vi "main.vi"() -> ()   [LabVIEW 2019]
uses:
  <vilib>/Utility/sysdir.llb/System Directory Type.ctl
  <vilib>/LabVIEW Open Source Project/MQTT Client/Client class/Client.lvclass/Client.ctl
  <vilib>/LabVIEW Open Source Project/MQTT Connection/MQTT_Base/Base Class/MQTT_Base.lvclass/MQTT_Base.ctl
  <vilib>/LabVIEW Open Source Project/MQTT Control Packets/Control Packets/ControlPacket/QualityOfService -- enum.ctl
  <vilib>/LabVIEW Open Source Project/MQTT Control Packets/Control Packets/ControlPacket/ControlPacket.lvclass/ControlPacket.ctl
  <vilib>/LabVIEW Open Source Project/MQTT Control Packets/Control Packets/CONNECT/ConnectFlags -- cluster.ctl
  <vilib>/LabVIEW Open Source Project/Connection/Connection.TCP/Connection.TCP.lvclass
  C:/Program Files (x86)/National Instruments/LabVIEW 2019/vi.lib/LabVIEW Open Source Project/Connection/Connection/Connection.lvclass
  <vilib>/LabVIEW Open Source Project/MQTT Client/Client class/Client.lvclass
  C:/Program Files (x86)/National Instruments/LabVIEW 2019/vi.lib/LabVIEW Open Source Project/MQTT Connection/MQTT_Base/Base Class/MQTT_Base.lvclass
  <vilib>/LabVIEW Open Source Project/MQTT Control Packets/Control Packets/PUBLISH/PUBLISH.lvclass
  C:/Program Files (x86)/National Instruments/LabVIEW 2019/vi.lib/LabVIEW Open Source Project/MQTT Control Packets/Control Packets/ControlPacket/ControlPacket.lvclass
  <vilib>/LabVIEW Open Source Project/MQTT Connection/MQTT_Base/Base Class/MQTT_Base.lvclass
  <vilib>/LabVIEW Open Source Project/MQTT Control Packets/Control Packets/ControlPacket/ControlPacket.lvclass
  <vilib>/LabVIEW Open Source Project/MQTT Control Packets/Control Packets/CONNECT/CONNECT.lvclass
  <vilib>/LabVIEW Open Source Project/Connection/Connection.LocalQueue/Connection.LocalQueue.lvclass
  <vilib>/LabVIEW Open Source Project/Connection/Connection/Connection.lvclass
panel:
  out "msg":string
  in  "publish":bool
  out "mac":string
  out "last error":errorcluster
  out "Database":bool
  out "Time Stamp Control":timestamp format="%<%X\n%x>T"
  in  "Tab Control":T1(tab)
  in  "Listbox":i32(listbox)
  in  "Users allowed per Node":u16(ring) items=["Veiculo QXC-01"]
  in  "Add Button":bool
  in  "Nodes":i32(listbox)
  in  "Users":i32(listbox)
  out "Users":dbl
  out "Nodes":dbl
  in  "Employee List":i32(listbox)
  in  "Nodes Esp32":i32(listbox)
  in  "Broker Port":dbl=1883.0
  in  "Broker Address":string="broker.hivemq.com"
  in  "Connection":bool
  in  "Subscribe":bool
  in  "Settings Button":bool
  in  "Payroll Button":bool
  in  "Logs Button":bool
  in  "Nodes Button":bool
  in  "Employee Button":bool
  in  "Home Button":bool
  # "COMING SOON"
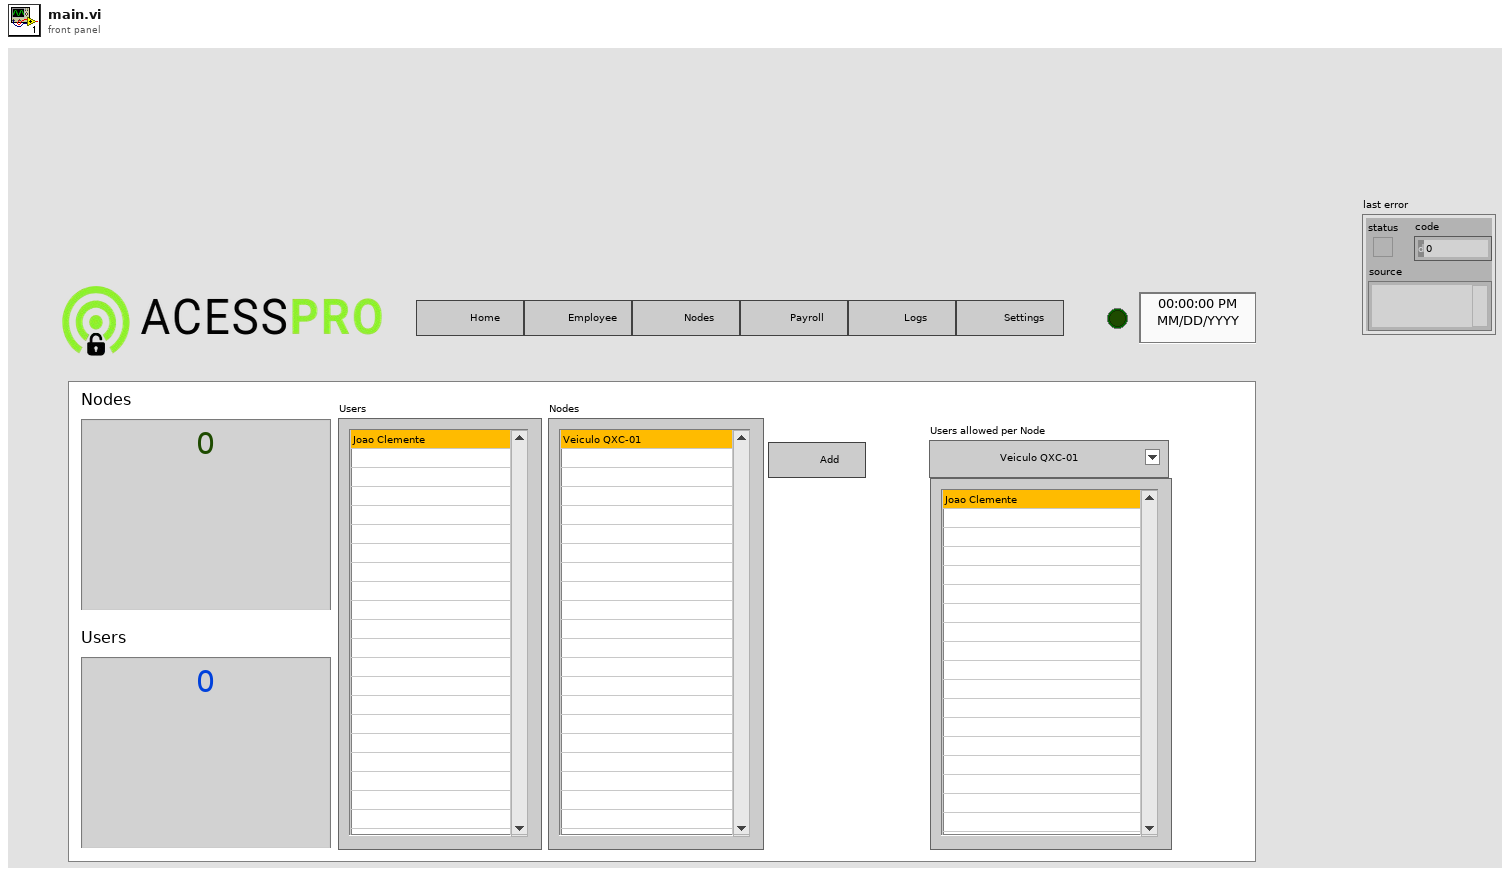
[diagram p1: front panel]
types:
  T1 = enum32{"Home", "Employee", "Nodes", "Payroll", "Logs", "Settings"}
  T2 = typedef "System Directory Type.ctl" = i32
  T3 = typedef "MQTT Client.lvlib/Client.lvclass/Public Events -- cluster.ctl" = cluster{"Connection Status":refnum<user-event>, "Connected":refnum<user-event>, "Application Message":refnum<user-event>}
  T4 = typedef "MQTT Base.lvlib/MQTT_Base.lvclass/Public Events -- cluster.ctl" = cluster{"Stop Event":refnum<user-event>, "Error Event":refnum<user-event>, "Inbound Message":refnum<user-event>}
  T5 = enum16{"open", "replace", "create", "open or create", "replace or create", "replace or create with confirmation"}
  T6 = typedef "MQTT_Control_Packets.lvlib/ControlPacket.lvclass/QualityOfService -- enum.ctl" = enum16{"0 (At Most Once)", "1 (At Least Once)", "2 (Exactly Once)"}
  T7 = cluster{"Will Topic":string, "Will Message":string, "Username":string, "Password":string}
  T8 = typedef "MQTT_Control_Packets.lvlib/CONNECT.lvclass/ConnectFlags -- cluster.ctl" = cluster{"Reserved":bool, "Clean Session":bool, "Will Flag":bool, "Will QoS 1":bool, "Will QoS 2":bool, "Will Retain":bool, "Password Flag":bool, "User Name Flag":bool}
  T9 = cluster{"regular expression":string, "Variant":variant}
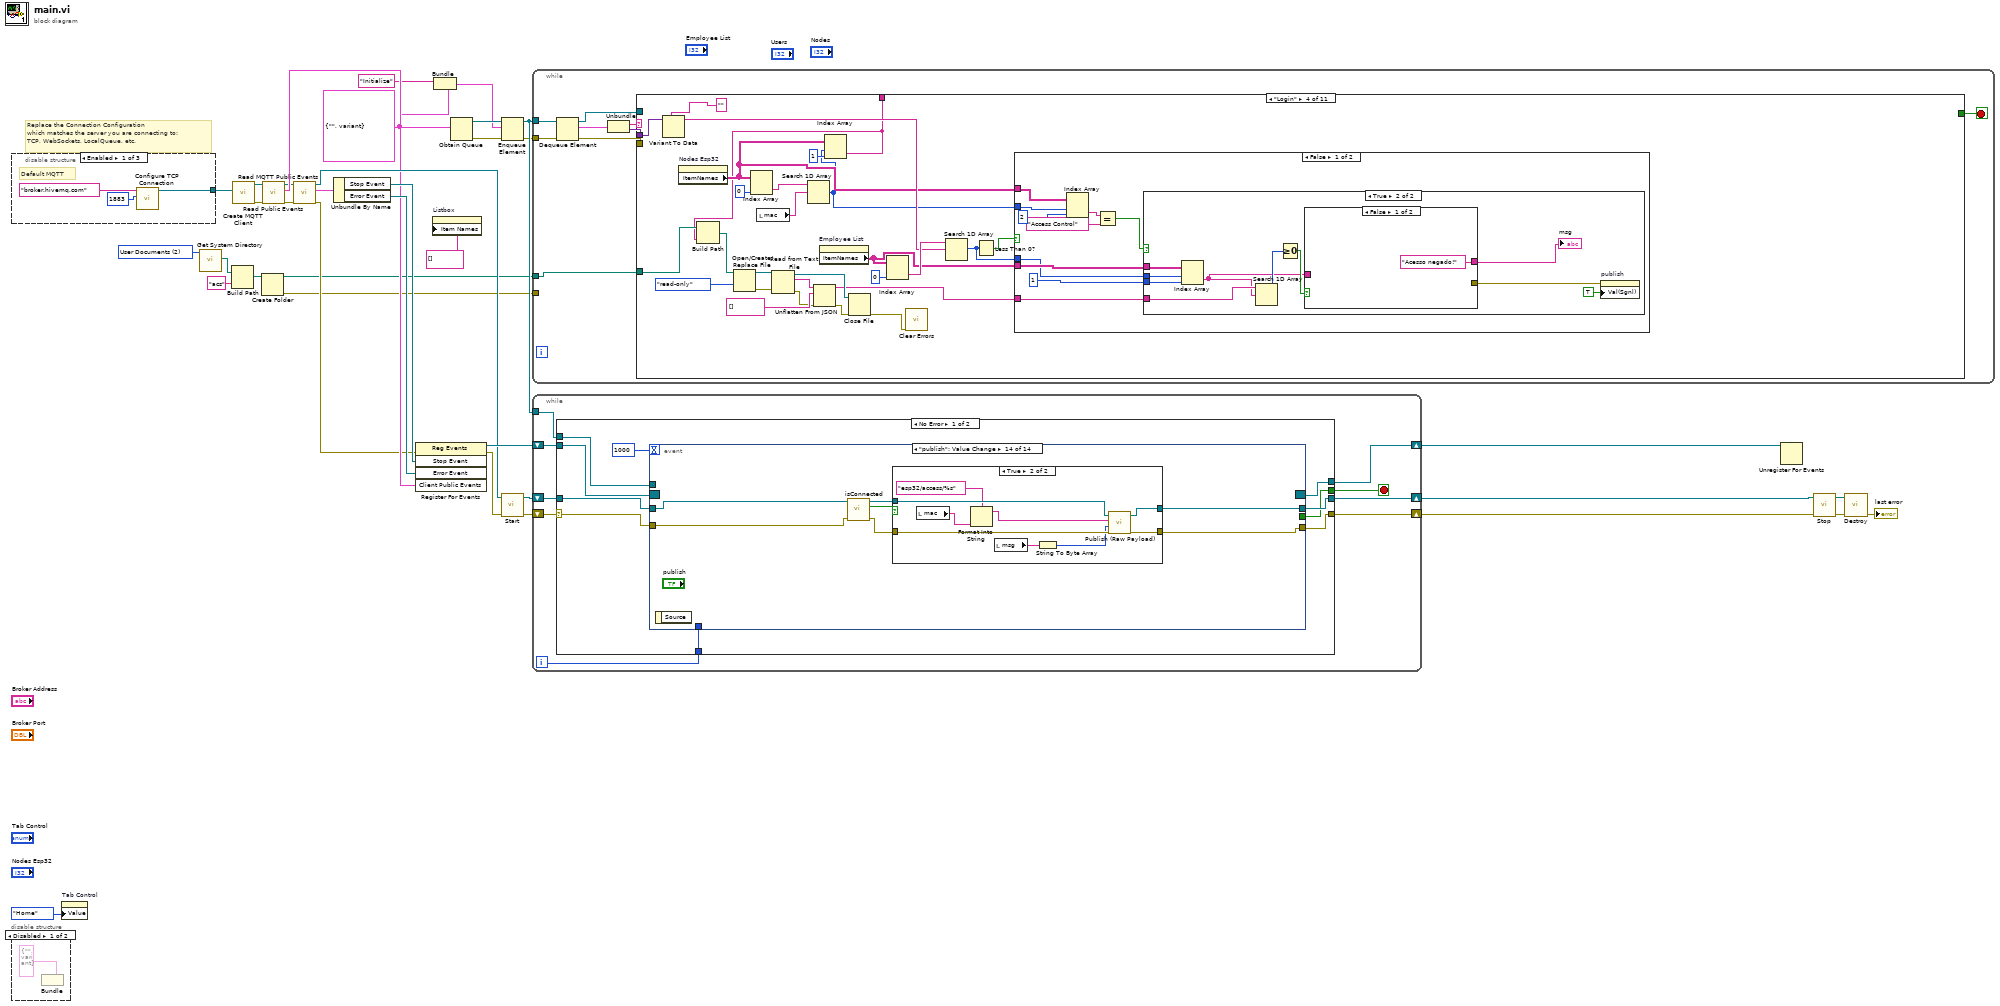
[diagram p0: block diagram]
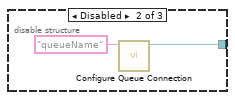
[diagram p3: hidden frame]
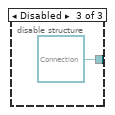
[diagram p4: hidden frame]
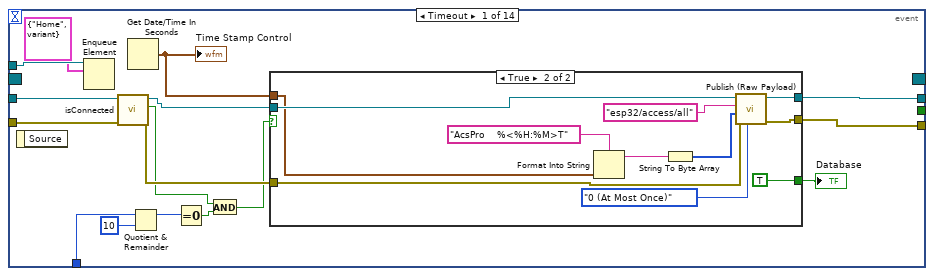
[diagram p5: hidden frame]
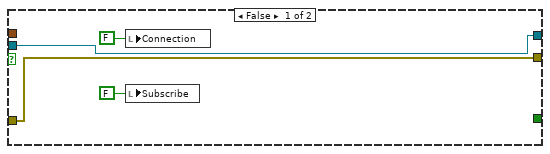
[diagram p6: hidden frame]
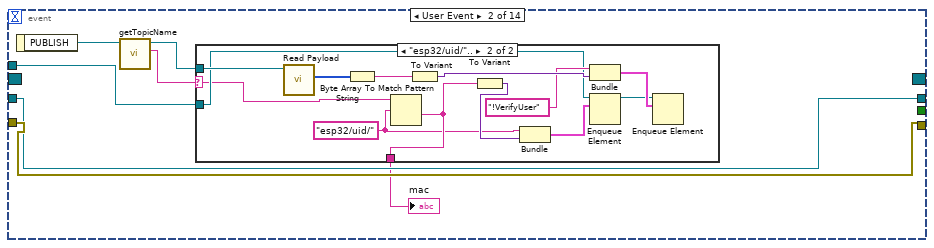
[diagram p7: hidden frame]
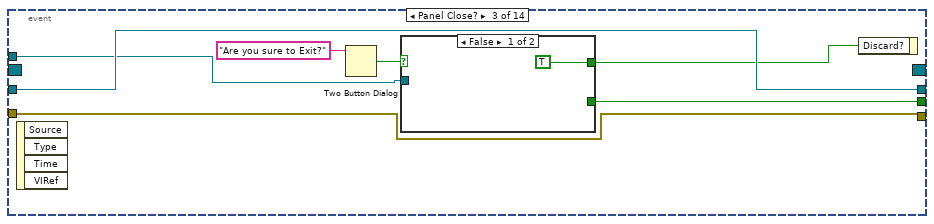
[diagram p9: hidden frame]
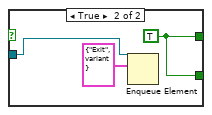
[diagram p10: hidden frame]
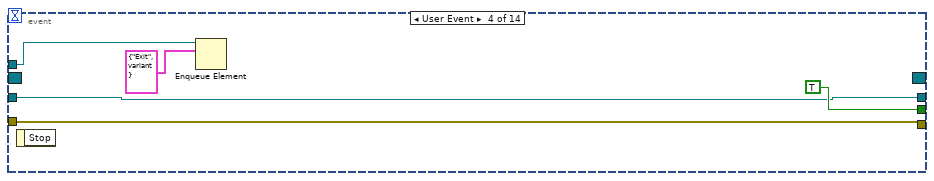
[diagram p11: hidden frame]
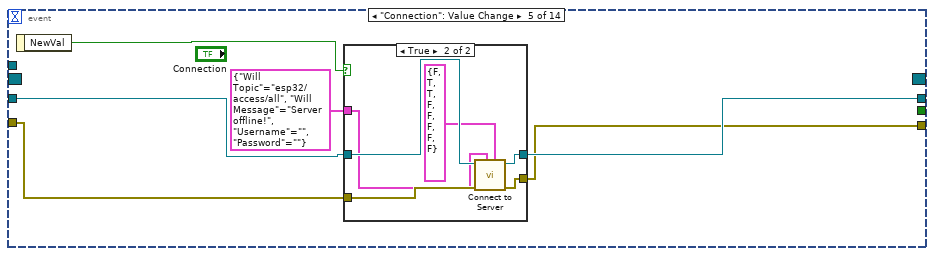
[diagram p12: hidden frame]
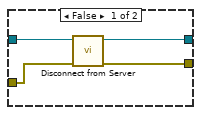
[diagram p13: hidden frame]
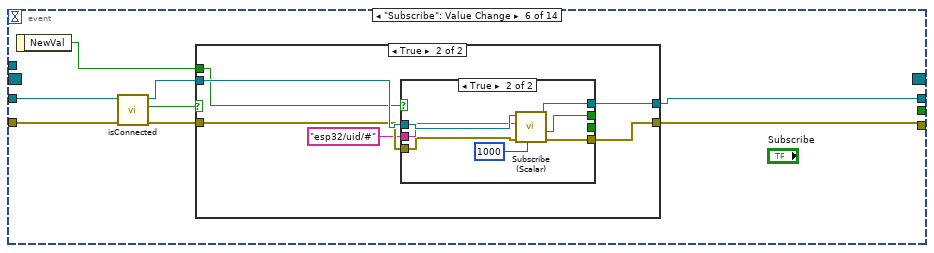
[diagram p14: hidden frame]
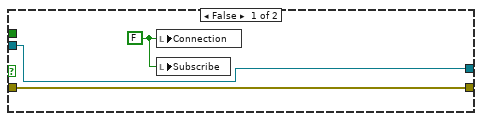
[diagram p15: hidden frame]
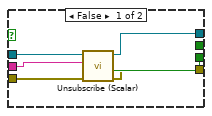
[diagram p16: hidden frame]
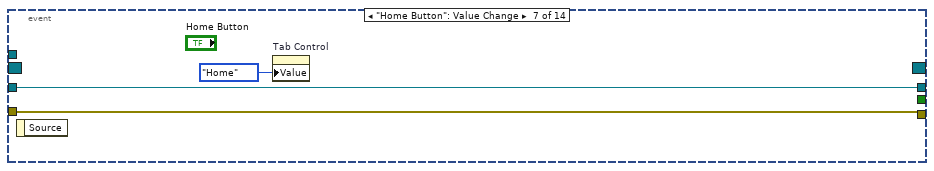
[diagram p17: hidden frame]
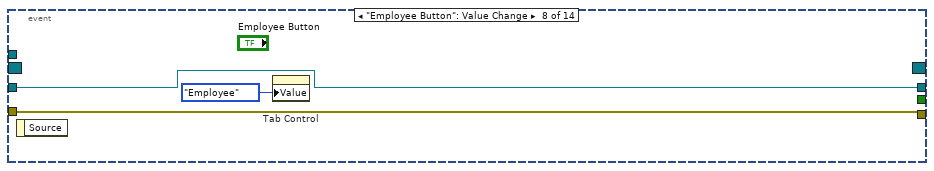
[diagram p18: hidden frame]
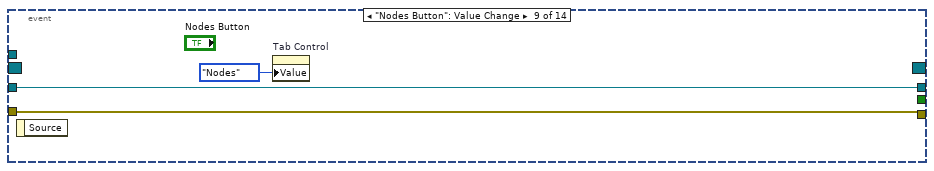
[diagram p19: hidden frame]
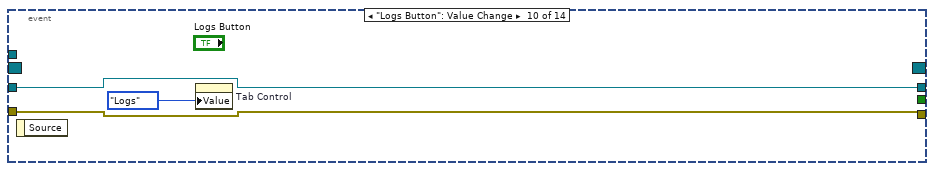
[diagram p20: hidden frame]
diagram:
  w4 = T2 2 items=["User Home"=0, "User Desktop"=1, "User Documents"=2, "User Application Data"=3, "User Preferences"=4, "User Temporary"=5, "Public Documents"=6, "Public Application Data"=7, "Public Preferences"=8, "Public Cache"=13, "System Core Libraries"=9, "System Installed Libraries"=10, "Application Files"=11, "Boot Volume Root"=12] ("system directory type")
  w11 = cluster{string, variant} {"", variant}
  # "Replace the Connection Configuration\nwhich matches the server you are connecting to:\nTCP, WebSockets, LocalQueue, etc."
  n1 = disable-structure shown="Enabled" {
    disable-tunnel: [w37 w41 refnum<class "Connection.lvclass"> refnum ("Connection Configuration")] -> w36
    frame Enabled {
      # "Default MQTT"
      n2 = call <vilib>:"Configure TCP Connection.vi"("remote port (80)"=u16 1883, "address (localhost)"="broker.hivemq.com") -> ("Connection.TCP"=w37:refnum<class "Connection.TCP.lvclass">)  [unwired: 8 in, 1 out]
    }
    frame Disabled {
      n3 = call <vilib>:"Configure Queue Connection.vi"("Queue Name"="queueName") -> ("Connection.LocalQueue"=w41:refnum<class "Connection.LocalQueue.lvclass">)  [unwired: 9 in, 1 out]
    }
    frame Disabled {
    }
  }
  n4 = disable-structure shown="Disabled" {
    frame Disabled {
      n5 = Bundle(cluster=cluster{string, variant} {"", variant} ("output cluster")) -> ()  [unwired: 2 in, 1 out]
    }
    frame Enabled {
    }
  }
  n6 = property on="Tab Control" class="TabCtl (strict)"("Value"=T1."Home" ("Tab Control")) -> ()  [unwired: 2 in, 2 out]
  n7 = call <vilib>:"Get System Directory.vi"("system directory type"=w4) -> ("system directory"=w6:path)  [unwired: 10 in]
  n8 = Build Path(base path=w6, name or relative path="acs") -> (appended path=w7:path)
  n9 = call <vilib>:"Create MQTT Client.vi"("Connection Configuration"=w36) -> ("error out"=w18:errorcluster, "Client out"=w16:refnum<class "Client.lvclass">)  [unwired: 9 in]
  n10 = Create Folder(path (use dialog)=w7) -> (created path=w2:path, error out=w3:errorcluster)  [unwired: 2 in, 1 out]
  n11 = call <vilib>:"Read Public Events.vi"("error in (no error)"=w18, "Client in"=w16) -> ("error out"=w19:errorcluster, "Client Public Events"=w21:T3, "Client out"=w17:refnum<class "Client.lvclass">)  [unwired: 7 in]
  n12 = call <vilib>:"Read MQTT Public Events.vi"("error in (no error)"=w19, "MQTT_Base in"=w17) -> ("error out"=w20:errorcluster, "MQTT Public Events"=w28:T4, "MQTT_Base out"=w23:refnum<class "Client.lvclass">)  [unwired: 7 in]
  n13 = Unbundle By Name(w28) -> ("Stop Event"=w26:refnum<user-event>, "Error Event"=w27:refnum<user-event>)
  n14 = register-events(error in=w20, w26, w27, w21) -> (reference out=w24:refnum<event-registration>, error out=w22:errorcluster)  [unwired: 1 in]
  n15 = property on="Listbox" class="LstBox (strict)"("Item Names"=string[] []) -> ()  [unwired: 2 in, 2 out]
  n16 = Bundle(cluster=w11, "Initialize") -> (w9:cluster{string, variant})  [unwired: 1 in]
  n17 = Obtain Queue(element data type=w11) -> (queue out=w14:refnum<queue>, error out=w15:errorcluster)  [unwired: 4 in, 1 out]
  n18 = Enqueue Element(queue=w14, element=w9, error in (no error)=w15) -> (queue out=w13:refnum<queue>, error out=w12:errorcluster)  [unwired: 1 in, 1 out]
  n19 = call <vilib>:"Start.vi"("error in (no error)"=w22, "MQTT_Base in"=w23) -> ("error out"=w34:errorcluster, "MQTT_Base out"=w33:refnum<class "Client.lvclass">)  [unwired: 7 in, 1 out]
  n20 = while {
    tunnel: w13 -> [w52]
    tunnel: w12 -> [w51]
    tunnel: w3 -> [_]
    tunnel: w2 -> [w44]
    stop <- w45 stop-if-true
    n21 = Dequeue Element(queue=w52, error in (no error)=w51) -> (queue out=w49:refnum<queue>, element=w50:cluster{string, variant}, error out=w48:errorcluster)  [unwired: 1 in, 1 out]
    n22 = Unbundle(w50) -> (w47:string, w46:variant)
    n23 = case shown="\"Login\"" w47 {
      tunnel: w49 -> [_ _ _ _ _ w183 w185 w202 _ _ _]
      tunnel: w48 -> [_ _ _ _ _ _ _ _ _ _ _]
      tunnel: w46 -> [_ _ _ w141 _ w179 w184 w201 w222 w245 _]
      tunnel: [FALSE _ _ _ _ _ _ _ _ _ TRUE] -> w45
      tunnel: w44 -> [_ w68 w75 w129 _ _ _ _ _ _ _]
      tunnel: [_ _ _ w128 _ _ _ _ _ _ _] -> _
      frame Default {
      }
      frame "Home" {
        w71 = 1 ("disabled index (col)")
        n24 = property on="Nodes Esp32" class="MCListbox (strict)"() -> ("ItemNames"=w72:string[][])  [unwired: 2 in, 2 out]
        n25 = List Folder(path=w68) -> (filenames=w69:string[])  [unwired: 3 in, 3 out]
        n26 = property on="Employee List" class="MCListbox (strict)"() -> ("ItemNames"=w74:string[][])  [unwired: 2 in, 2 out]
        n27 = property on="Users allowed per Node" class="Ring (strict)"("Strings []"=w69) -> ()  [unwired: 2 in, 2 out]
        n28 = Index Array(array=w74, index (col)=w71) -> (element=w54:string[])  [unwired: 1 in]
        n29 = Index Array(array=w72, index (col)=w71) -> (element=w55:string[])  [unwired: 1 in]
        n30 = Array Size(array=w54) -> (size(s)=→"Users":i32)
        n31 = Array Size(array=w55) -> (size(s)=→"Nodes":i32)
        n32 = property on="Users allowed per Node" class="Ring (strict)"() -> ("RingText.Text"=w67:string)  [unwired: 2 in, 2 out]
        n33 = Build Path(base path=w68, name or relative path=w67) -> (appended path=w66:path)
        n34 = property on="Nodes" class="LstBox (strict)"("Item Names"=w55) -> ()  [unwired: 2 in, 2 out]
        n35 = property on="Users" class="LstBox (strict)"("Item Names"=w54) -> ()  [unwired: 2 in, 2 out]
        n36 = Open/Create/Replace File(file path (use dialog)=w66, access (0:read/write)=enum16{"read/write", "read-only", "write-only"}."read-only") -> (refnum out=w63:refnum<file>, error out=w64:errorcluster)  [unwired: 4 in, 1 out]
        n37 = Read from Text File(file (use dialog)=w63, error in=w64) -> (refnum out=w61:refnum<file>, text=w60:string, error out=w62:errorcluster)  [unwired: 2 in, 1 out]
        n38 = Close File(refnum=w61, error in=w62) -> (error out=w58:errorcluster)  [unwired: 1 out]
        n39 = Unflatten From JSON(JSON string=w60, type and defaults=string[] [], error in (no error)=w58) -> (value=w56:string[], error out=w57:errorcluster)  [unwired: 4 in]
        n40 = call <vilib>:"Clear Errors.vi"("error in (no error)"=w57) -> ()  [unwired: 5 in, 2 out]
        n41 = property on="Listbox" class="LstBox (strict)"("Item Names"=w56) -> ()  [unwired: 2 in, 2 out]
      }
      frame "TreeAcessControl" {
        w81 = -1 ("y")
        n42 = property on="Nodes" class="LstBox (strict)"() -> ("Value"=w82:i32)  [unwired: 2 in, 2 out]
        n43 = property on="Users" class="LstBox (strict)"() -> ("Value"=w83:i32)  [unwired: 2 in, 2 out]
        n44 = Greater?(x=w83, y=w81) -> (0:w80:bool)
        n45 = Greater?(x=w82, y=w81) -> (0:w79:bool)
        n46 = property on="Users" class="LstBox (strict)"() -> ("Item Names"=w84:string[])  [unwired: 2 in, 2 out]
        n47 = property on="Nodes" class="LstBox (strict)"() -> ("Item Names"=w85:string[])  [unwired: 2 in, 2 out]
        n48 = Index Array(array=w85, index=w82) -> (element=w77:string)
        n49 = Index Array(array=w84, index=w83) -> (element=w76:string)
        n50 = And(x=w80, y=w79) -> (x .and. y?=w78:bool)
        n51 = case shown="True" w78 {
          tunnel: w77 -> [_ w99]
          tunnel: w76 -> [_ w92]
          tunnel: w75 -> [_ w100]
          frame False {
            n52 = One Button Dialog(message="User and Node must be selected!") -> ()  [unwired: 1 in, 1 out]
          }
          frame True {
            n53 = Build Path(base path=w100, name or relative path=w99) -> (appended path=w87:path)
            n54 = Open/Create/Replace File(file path (use dialog)=w87, operation (0:open)=T5."open or create") -> (refnum out=w96:refnum<file>, error out=w97:errorcluster)  [unwired: 4 in, 1 out]
            n55 = Read from Text File(file (use dialog)=w96, error in=w97) -> (refnum out=w94:refnum<file>, text=w89:string, error out=w93:errorcluster)  [unwired: 2 in, 1 out]
            n56 = Unflatten From JSON(JSON string=w89, type and defaults=string[] [] ("appended array")) -> (value=w91:string[], error out=w90:errorcluster)  [unwired: 5 in]
            n57 = for {
              tunnel: w92 -> [w118]
              tunnel: [w117] -> w95
              tunnel: w91 -> [w116] mode=indexing
              tunnel: w90 -> [_]
              stop <- w117 stop-if-true
              n58 = Equal?(x=w116, y=w118) -> (x = y?=w117:bool)
            }
            n59 = case shown="False" w95 {
              tunnel: w94 -> [w109 w115]
              tunnel: w93 -> [w108 w114]
              tunnel: w92 -> [w113 _]
              tunnel: w91 -> [w112 _]
              tunnel: [w101 _] -> _
              frame False {
                n60 = Close File(refnum=w109, error in=w108) -> (path=w107:path)  [unwired: 1 out]
                n61 = Build Array (concatenate)(w112, w113) -> (w111:string[])
                n62 = Flatten To JSON(anything=w111) -> (JSON string=w110:string)  [unwired: 2 in, 1 out]
                n63 = Open/Create/Replace File(file path (use dialog)=w107, operation (0:open)=T5."replace") -> (refnum out=w105:refnum<file>, error out=w104:errorcluster)  [unwired: 4 in, 1 out]
                n64 = Write to Text File(file (use dialog)=w105, text=w110, error in=w104) -> (refnum out=w102:refnum<file>, error out=w103:errorcluster)  [unwired: 1 in, 1 out]
                n65 = Close File(refnum=w102, error in=w103) -> (error out=w101:errorcluster)  [unwired: 1 out]
              }
              frame True {
                # "Ja existe"
                n66 = Close File(refnum=w115, error in=w114) -> ()  [unwired: 2 out]
              }
            }
          }
        }
      }
      frame "Login" {
        n67 = Variant To Data(type="", Variant=w141) -> (data=w137:string)  [unwired: 1 in, 1 out]
        n68 = property on="Nodes Esp32" class="MCListbox (strict)"() -> ("ItemNames"=w133:string[][])  [unwired: 2 in, 2 out]
        n69 = Index Array(array=w133, index (col)=0 ("disabled index (col)")) -> (element=w144:string[])  [unwired: 1 in]
        n70 = local read "mac"() -> (w143:string)
        n71 = Search 1D Array(1D array=w144, element=w143) -> (index of element=w132:i32)  [unwired: 1 in]
        n72 = property on="Employee List" class="MCListbox (strict)"() -> ("ItemNames"=w135:string[][])  [unwired: 2 in, 2 out]
        n73 = Index Array(array=w133, index (row)=w132, index (col)=1 ("disabled index (col)")) -> (element=w128:string)
        n74 = Build Path(base path=w129, name or relative path=w128) -> (appended path=w130:path)
        n75 = Open/Create/Replace File(file path (use dialog)=w130, access (0:read/write)=enum16{"read/write", "read-only", "write-only"}."read-only") -> (refnum out=w126:refnum<file>, error out=w127:errorcluster)  [unwired: 4 in, 1 out]
        n76 = Read from Text File(file (use dialog)=w126, error in=w127) -> (refnum out=w121:refnum<file>, text=w125:string, error out=w123:errorcluster)  [unwired: 2 in, 1 out]
        n77 = Unflatten From JSON(JSON string=w125, type and defaults=string[] [] ("text"), error in (no error)=w123) -> (value=w120:string[], error out=w122:errorcluster)  [unwired: 4 in]
        n78 = Close File(refnum=w121, error in=w122) -> (error out=w119:errorcluster)  [unwired: 1 out]
        n79 = Index Array(array=w135, index (col)=0 ("disabled index (col)")) -> (element=w138:string[])  [unwired: 1 in]
        n80 = call <vilib>:"Clear Errors.vi"("error in (no error)"=w119) -> ()  [unwired: 5 in, 2 out]
        n81 = Search 1D Array(1D array=w138, element=w137) -> (index of element=w134:i32)  [unwired: 1 in]
        n82 = Less Than 0?(x=w134) -> (x < 0?=w136:bool)
        n83 = case shown="False" w136 {
          tunnel: w135 -> [w155 _]
          tunnel: w134 -> [w153 _]
          tunnel: w133 -> [w152 _]
          tunnel: w132 -> [w150 _]
          tunnel: w120 -> [w146 _]
          frame False {
            n84 = Index Array(array=w152, index (row)=w150, index (col)=2 ("disabled index (col)")) -> (element=w149:string)
            n85 = Equal?(x=w149, y="Access Control") -> (x = y?=w147:bool)
            n86 = case shown="True" w147 {
              tunnel: w155 -> [_ w165]
              tunnel: 1 ("disabled index (col)") -> [_ w164]
              tunnel: w153 -> [_ w163]
              tunnel: w146 -> [_ w162]
              frame False {
              }
              frame True {
                n87 = Index Array(array=w165, index (row)=w163, index (col)=w164) -> (element=w158:string)
                n88 = Search 1D Array(1D array=w162, element=w158) -> (index of element=w161:i32)  [unwired: 1 in]
                n89 = Greater Or Equal To 0?(x=w161) -> (x >= 0?=w160:bool)
                n90 = case shown="False" w160 {
                  tunnel: w158 -> [_ w170]
                  tunnel: ["Acesso negado!" w169] -> w157
                  tunnel: [_ w168] -> w156
                  frame False {
                  }
                  frame True {
                    n91 = Format Into String(format string="%s seu acesso está autorizado!", w170) -> (resulting string=w169:string, error out=w168:errorcluster)  [unwired: 2 in]
                  }
                }
                "msg" <- w157
                n92 = property on="publish" class="Bool (strict)"(error in=w156, "Val(Sgnl)"=TRUE ("Value (Signaling)")) -> ()  [unwired: 1 in, 2 out]
              }
            }
          }
          frame True {
            # "não encontrou"
          }
        }
      }
      frame "Initialize" {
        n93 = property on="Connection" class="Bool (strict)"("Val(Sgnl)"=TRUE ("Value (Signaling)")) -> (error out=w173:errorcluster)  [unwired: 2 in, 1 out]
        n94 = flat-sequence {
          tunnel: w173 -> [w177]
          tunnel: [w177] -> w172
          tunnel: [w176] -> w171
          frame #0 {
            n95 = Wait (ms)(milliseconds to wait=u32 3000) -> ()  [unwired: 1 out]
            n96 = call <vilib>:"Set Busy.vi"() -> ("error out"=w176:errorcluster)  [unwired: 10 in, 1 out]
          }
        }
        n97 = call <vilib>:"Unset Busy.vi"("error in (no error)"=w171) -> ()  [unwired: 10 in, 1 out]
        n98 = property on="Subscribe" class="Bool (strict)"(error in=w172, "Val(Sgnl)"=TRUE ("Value (Signaling)")) -> ()  [unwired: 1 in, 2 out]
      }
      frame "esp32/uid/" {
        n99 = Bundle(cluster=cluster{string, variant} {"", variant} ("element"), "!VerifyNode", w179) -> (w182:cluster{string, variant})
        n100 = Enqueue Element At Opposite End(queue=w183, element=w182) -> ()  [unwired: 2 in, 3 out]
      }
      frame "!VerifyNode" {
        n101 = property on="Nodes Esp32" class="MCListbox (strict)"() -> ("ItemNames"=w190:string[][])  [unwired: 2 in, 2 out]
        n102 = Index Array(array=w190, index (col)=0 ("disabled index (col)")) -> (element=w188:string[])  [unwired: 1 in]
        n103 = Variant To Data(type="", Variant=w184) -> (data=w187:string)  [unwired: 1 in, 1 out]
        n104 = for {
          tunnel: w188 -> [w198] mode=indexing
          tunnel: w187 -> [w197]
          tunnel: [w196] -> w186
          stop <- w196 stop-if-true
          n105 = Equal?(x=w197, y=w198) -> (x = y?=w196:bool)
        }
        n106 = case shown="False" w186 {
          tunnel: w185 -> [w195 _]
          tunnel: w184 -> [w192 _]
          frame False {
            n107 = Bundle("!CreateNode", w192) -> (w194:cluster{string, variant})  [unwired: 1 in]
            n108 = Enqueue Element(queue=w195, element=w194) -> ()  [unwired: 2 in, 3 out]
          }
          frame True {
          }
        }
      }
      frame "!VerifyUser" {
        n109 = property on="Employee List" class="MCListbox (strict)"() -> ("ItemNames"=w200:string[][])  [unwired: 2 in, 2 out]
        n110 = Index Array(array=w200, index (col)=0 ("disabled index (col)")) -> (element=w205:string[])  [unwired: 1 in]
        n111 = Variant To Data(type="", Variant=w201) -> (data=w204:string)  [unwired: 1 in, 1 out]
        n112 = for {
          tunnel: w205 -> [w218] mode=indexing
          tunnel: w204 -> [w217]
          tunnel: [w216] -> w203
          stop <- w216 stop-if-true
          n113 = Equal?(x=w217, y=w218) -> (x = y?=w216:bool)
        }
        n114 = case shown="True" w203 {
          tunnel: w202 -> [w211 w215]
          tunnel: w201 -> [w208 w212]
          tunnel: "Login" -> [_ w213]
          frame False {
            n115 = Bundle("!CreateUser", w208) -> (w210:cluster{string, variant})  [unwired: 1 in]
            n116 = Enqueue Element(queue=w211, element=w210) -> ()  [unwired: 2 in, 3 out]
          }
          frame True {
            n117 = Bundle(w213, w212) -> (w214:cluster{string, variant})  [unwired: 1 in]
            n118 = Enqueue Element(queue=w215, element=w214) -> ()  [unwired: 2 in, 3 out]
          }
        }
      }
      frame "!CreateNode" {
        w221 = "The system detect new\nnode running on cloud.\n\nDo you want to insert?\n\nNode ID: %s" ("format string")
        n119 = Variant To Data(type=w221, Variant=w222) -> (data=w219:string)  [unwired: 1 in, 1 out]
        n120 = Format Into String(format string=w221, w219) -> (resulting string=w223:string)  [unwired: 2 in, 1 out]
        n121 = Two Button Dialog(message=w223) -> (T button?=w220:bool)  [unwired: 2 in]
        n122 = case shown="True" w220 {
          tunnel: w219 -> [_ w229]
          frame False {
          }
          frame True {
            n123 = call "Insert New Node"() -> ("Description"=w225:string, "Is Acess Control?"=w227:bool, "Location"=w228:string, "OK"=w224:bool)  [unwired: 15 in, 1 out]
            n124 = property on="Tab Control" class="TabCtl (strict)"("Value"=T1."Nodes" ("Tab Control")) -> ()  [unwired: 2 in, 2 out]
            n125 = case shown="True" w224 {
              tunnel: w229 -> [_ w239]
              tunnel: w228 -> [_ w238]
              tunnel: w227 -> [_ w237]
              tunnel: "Access Control" ("Location") -> [_ w236]
              tunnel: w225 -> [_ w232]
              frame False {
              }
              frame True {
                n126 = Select(t=w236, s=w237, f="Clock In" ("Location")) -> (s? t:f=w234:string)
                n127 = property on="Nodes Esp32" class="MCListbox (strict)"() -> ("ItemNames"=w241:string[][])  [unwired: 2 in, 2 out]
                n128 = Build Array(w239, w238, w234, "OK" ("element"), w232) -> (w231:string[])
                n129 = Insert Into Array(array=w241, new element=w231) -> (w240:string[][])  [unwired: 2 in]
                n130 = property on="Nodes Esp32" class="MCListbox (strict)"("ItemNames"=w240) -> ()  [unwired: 2 in, 2 out]
              }
            }
          }
        }
      }
      frame "!CreateUser" {
        w244 = "The system detect new\nuser\n\nDo you want to insert?\n\nUser ID: %s" ("format string")
        n131 = Variant To Data(type=w244, Variant=w245) -> (data=w242:string)  [unwired: 1 in, 1 out]
        n132 = Format Into String(format string=w244, w242) -> (resulting string=w246:string)  [unwired: 2 in, 1 out]
        n133 = Two Button Dialog(message=w246) -> (T button?=w243:bool)  [unwired: 2 in]
        n134 = case shown="True" w243 {
          tunnel: w242 -> [_ w251]
          frame False {
          }
          frame True {
            n135 = call "Insert New User"() -> ("role"=w248:string, "e-mail"=w249:string, "Name"=w250:string, "OK"=w247:bool)  [unwired: 15 in, 1 out]
            n136 = property on="Tab Control" class="TabCtl (strict)"("Value"=T1."Employee" ("Tab Control")) -> ()  [unwired: 2 in, 2 out]
            n137 = case shown="True" w247 {
              tunnel: w251 -> [_ w259]
              tunnel: w250 -> [_ w257]
              tunnel: w249 -> [_ w254]
              tunnel: w248 -> [_ w253]
              frame False {
              }
              frame True {
                n138 = Build Array(w259, w257, w254, w253) -> (w258:string[])
                n139 = property on="Employee List" class="MCListbox (strict)"() -> ("ItemNames"=w256:string[][])  [unwired: 2 in, 2 out]
                n140 = Insert Into Array(array=w256, new element=w258) -> (w255:string[][])  [unwired: 2 in]
                n141 = property on="Employee List" class="MCListbox (strict)"("ItemNames"=w255) -> ()  [unwired: 2 in, 2 out]
              }
            }
          }
        }
      }
      frame "Exit" {
      }
    }
  }
  n142 = while {
    shift-right: [w268] -> w25
    shift-left: w24 -> [w269]
    shift-right: [w265] -> w30
    shift-left: w33 -> [w266]
    shift-right: [w267] -> w32
    shift-left: w34 -> [w263]
    tunnel: w13 -> [w262]
    i -> [w261]
    stop <- w264 stop-if-true
    n143 = case shown="No Error" w263 {
      selector: w263 -> [w272 w435]
      tunnel: w269 -> [w279 w434]
      tunnel: [w278 w433] -> w268
      tunnel: [w277 w437] -> w267
      tunnel: w266 -> [w275 w438]
      tunnel: [w274 w440] -> w265
      tunnel: [w273 w436] -> w264
      tunnel: w262 -> [w271 _]
      tunnel: w261 -> [w270 _]
      frame No Error {
        n144 = event shown="[13] \"publish\": Value Change" {
          selector: w279 -> [_ _ _ _ _ _ _ _ _ _ _ _ _ _]
          dyn-events: [_ _ _ _ _ _ _ _ _ _ _ _ _ _] -> w278
          timeout: 1000 -> [_ _ _ _ _ _ _ _ _ _ _ _ _ _]
          tunnel: w272 -> [w291 w316 w335 w346 w348 w368 w393 w397 w401 w404 w406 w409 w411 w420]
          tunnel: [w294 w316 w335 w346 w349 w369 w393 w397 w401 w404 w406 w409 w411 w415] -> w277
          tunnel: [_ _ w337 TRUE _ _ _ _ _ _ _ _ _ _] -> w273
          tunnel: w275 -> [w293 w315 w336 w344 w352 w367 w394 w396 w400 w403 w405 w408 w412 w421]
          tunnel: [w295 w315 w336 w344 w350 w370 w394 w396 w400 w403 w405 w408 w412 w417] -> w274
          tunnel: w271 -> [w288 w312 w334 w343 _ _ _ _ _ _ _ _ w414 _]
          tunnel: w270 -> [w285 _ _ _ _ _ _ _ _ _ _ _ _ _]
          event Timeout {
            n145 = event-data() -> ()  [unwired: 1 in, 1 out]
            n146 = Enqueue Element(queue=w288, element=cluster{string, variant} {"Home", variant}) -> ()  [unwired: 2 in, 3 out]
            n147 = call <vilib>:"isConnected.vi"("error in (no error)"=w291, "Client in"=w293) -> ("error out"=w290:errorcluster, "connected"=w281:bool, "Client out"=w292:refnum<class "Client.lvclass">)  [unwired: 7 in]
            n148 = Get Date/Time In Seconds() -> (seconds since 1Jan1904=w289:timestamp)
            "Time Stamp Control" <- w289
            n149 = Quotient & Remainder(x=w285, y=10) -> (x-y*floor(x/y)=w283:i32)  [unwired: 1 out]
            n150 = Equal To 0?(x=w283) -> (x = 0?=w282:bool)
            n151 = And(x=w281, y=w282) -> (x .and. y?=w280:bool)
            n152 = case shown="True" w280 {
              tunnel: [w299 w306] -> w295
              tunnel: [w298 w307] -> w294
              tunnel: w292 -> [w299 w310]
              tunnel: w290 -> [w298 w309]
              tunnel: w289 -> [_ w303]
              tunnel: [_ TRUE ("Database")] -> w286
              frame False {
                n153 = local write "Connection"(FALSE ("Connection")) -> ()
                n154 = local write "Subscribe"(FALSE) -> ()
              }
              frame True {
                n155 = Format Into String(format string="AcsPro    %<%H:%M>T", w303) -> (resulting string=w302:string)  [unwired: 2 in, 1 out]
                n156 = String To Byte Array(string=w302) -> (unsigned byte array=w301:u8[])
                n157 = call <vilib>:"Publish (Raw Payload).vi"("QoS"=QualityOfService_--_enum."0 (At Most Once)", "error in (no error)"=w309, "Binary Payload"=w301, "Topic Name"="esp32/access/all" ("Topic Name (empty: Payload name)"), "Client in"=w310) -> ("error out"=w307:errorcluster, "Client out"=w306:refnum<class "Client.lvclass">)  [unwired: 4 in, 1 out]
              }
            }
            "Database" <- w286
          }
          event User Event {
            n158 = event-data() -> ("PUBLISH"=w317:refnum<class "PUBLISH.lvclass">)  [unwired: 1 in]
            n159 = call <vilib>:"getTopicName.vi"("PUBLISH in"=w317) -> ("Topic"=w313:string, "PUBLISH out"=w314:refnum<class "PUBLISH.lvclass">)  [unwired: 8 in, 1 out]
            n160 = case shown="\"esp32/uid/\".." w313 {
              selector: w313 -> [_ w320]
              tunnel: w314 -> [_ w330]
              tunnel: w312 -> [_ w324]
              tunnel: [_ w319] -> w311
              frame Default {
              }
              frame "esp32/uid/".. {
                w318 = "esp32/uid/" ("regular expression")
                n161 = call <vilib>:"Read Payload.vi"("ControlPacket in"=w330) -> ("Payload"=w329:u8[])  [unwired: 9 in, 1 out]
                n162 = Byte Array To String(unsigned byte array=w329) -> (string=w328:string)
                n163 = Match Pattern(string=w320, regular expression=w318) -> (after substring=w319:string)  [unwired: 1 in, 3 out]
                n164 = To Variant(anything=w328) -> (Variant=w327:variant)
                n165 = To Variant(anything=w319) -> (Variant=w321:variant)
                n166 = Bundle("regular expression"=w318, "Variant"=w321) -> (w322:T9)  [unwired: 1 in]
                n167 = Bundle("!VerifyUser", "Variant"=w327) -> (w326:cluster{string, "Variant":variant})  [unwired: 1 in]
                n168 = Enqueue Element(queue=w324, element=w322) -> (queue out=w323:refnum<queue>)  [unwired: 2 in, 2 out]
                n169 = Enqueue Element(queue=w323, element=w326) -> ()  [unwired: 2 in, 3 out]
              }
            }
            "mac" <- w311
          }
          event Panel Close? {
            n170 = event-data() -> ()  [unwired: 1 in, 4 out]
            n171 = Two Button Dialog(message="Are you sure to Exit?") -> (T button?=w332:bool)  [unwired: 2 in]
            n172 = case shown="False" w332 {
              tunnel: [_ w339] -> w337
              tunnel: w334 -> [_ w341]
              tunnel: [TRUE w339] -> w331
              frame False {
              }
              frame True {
                w339 = TRUE
                n173 = Enqueue Element(queue=w341, element=cluster{string, variant} {"Exit", variant}) -> ()  [unwired: 2 in, 3 out]
              }
            }
            n174 = event-data("Discard?"=w331) -> ()  [unwired: 1 in, 1 out]
          }
          event User Event {
            n175 = event-data() -> ()  [unwired: 1 in, 1 out]
            n176 = Enqueue Element(queue=w343, element=cluster{string, variant} {"Exit", variant}) -> ()  [unwired: 2 in, 3 out]
          }
          event "Connection": Value Change {
            n177 = event-data() -> ("NewVal"=w351:bool)  [unwired: 1 in]
            n178 = case shown="True" w351 {
              tunnel: w352 -> [w356 w362]
              tunnel: [w355 w359] -> w350
              tunnel: [w354 w360] -> w349
              tunnel: w348 -> [w353 w361]
              tunnel: T7 {"Will Topic"="esp32/access/all", "Will Message"="Server offline!", "Username"="", "Password"=""} ("Payload") -> [_ w357]
              frame False {
                n179 = call <vilib>:"Disconnect from Server.vi"("error in (no error)"=w353, "Client in"=w356) -> ("error out"=w354:errorcluster, "Client out"=w355:refnum<class "Client.lvclass">)  [unwired: 7 in, 1 out]
              }
              frame True {
                n180 = call <vilib>:"Connect to Server.vi"("Connect Flags"=T8 {"Reserved"=FALSE, "Clean Session"=TRUE, "Will Flag"=TRUE, "Will QoS 1"=FALSE, "Will QoS 2"=FALSE, "Will Retain"=FALSE, "Password Flag"=FALSE, "User Name Flag"=FALSE}, "Payload"=w357, "error in (no error)"=w361, "Client in"=w362) -> ("error out"=w360:errorcluster, "Client out"=w359:refnum<class "Client.lvclass">)  [unwired: 4 in, 2 out]
              }
            }
          }
          event "Subscribe": Value Change {
            n181 = event-data() -> ("NewVal"=w363:bool)  [unwired: 1 in]
            n182 = call <vilib>:"isConnected.vi"("error in (no error)"=w368, "Client in"=w367) -> ("error out"=w365:errorcluster, "connected"=w364:bool, "Client out"=w366:refnum<class "Client.lvclass">)  [unwired: 7 in]
            n183 = case shown="True" w364 {
              tunnel: [w373 w379] -> w370
              tunnel: [w372 w378] -> w369
              tunnel: w366 -> [w373 w377]
              tunnel: w365 -> [w372 w376]
              tunnel: w363 -> [_ w374]
              frame False {
                w371 = FALSE ("Connection")
                n184 = local write "Connection"(w371) -> ()
                n185 = local write "Subscribe"(w371) -> ()
              }
              frame True {
                n186 = case shown="True" w374 {
                  tunnel: [w382 w391] -> w379
                  tunnel: [w380 w388] -> w378
                  tunnel: w377 -> [w385 w392]
                  tunnel: w376 -> [w384 w389]
                  tunnel: "esp32/uid/#" ("Topic Name (empty: Payload name)") -> [w383 w390]
                  tunnel: [_ w387] -> _
                  tunnel: [w381 _] -> _
                  frame False {
                    n187 = call <vilib>:"Unsubscribe (Scalar).vi"("error in (no error)"=w384, "Topic Filter"=w383, "Client in"=w385) -> ("error out"=w380:errorcluster, "Ack"=w381:bool, "Client out"=w382:refnum<class "Client.lvclass">)  [unwired: 6 in]
                  }
                  frame True {
                    n188 = call <vilib>:"Subscribe (Scalar).vi"("timeout (1000ms)"=1000 ("timeout (100ms)"), "error in (no error)"=w389, "Topic Filter"=w390, "Client in"=w392) -> ("error out"=w388:errorcluster, "Ack"=w387:bool, "Client out"=w391:refnum<class "Client.lvclass">)  [unwired: 5 in]
                  }
                }
              }
            }
          }
          event "Home Button": Value Change {
            n189 = event-data() -> ()  [unwired: 1 in, 1 out]
            n190 = property on="Tab Control" class="TabCtl (strict)"("Value"=T1."Home" ("Tab Control")) -> ()  [unwired: 2 in, 2 out]
          }
          event "Employee Button": Value Change {
            n191 = event-data() -> ()  [unwired: 1 in, 1 out]
            n192 = property on="Tab Control" class="TabCtl (strict)"("Value"=T1."Employee" ("Tab Control")) -> ()  [unwired: 2 in, 2 out]
          }
          event "Nodes Button": Value Change {
            n193 = event-data() -> ()  [unwired: 1 in, 1 out]
            n194 = property on="Tab Control" class="TabCtl (strict)"("Value"=T1."Nodes" ("Tab Control")) -> ()  [unwired: 2 in, 2 out]
          }
          event "Logs Button": Value Change {
            n195 = event-data() -> ()  [unwired: 1 in, 1 out]
            n196 = property on="Tab Control" class="TabCtl (strict)"("Value"=T1."Logs" ("Tab Control")) -> ()  [unwired: 2 in, 2 out]
          }
          event "Payroll Button": Value Change {
            n197 = event-data() -> ()  [unwired: 1 in, 1 out]
            n198 = property on="Tab Control" class="TabCtl (strict)"("Value"=T1."Payroll" ("Tab Control")) -> ()  [unwired: 2 in, 2 out]
          }
          event "Settings Button": Value Change {
            n199 = event-data() -> ()  [unwired: 1 in, 1 out]
            n200 = property on="Tab Control" class="TabCtl (strict)"("Value"=T1."Settings" ("Tab Control")) -> ()  [unwired: 2 in, 2 out]
          }
          event "Add Button": Value Change {
            n201 = event-data() -> ()  [unwired: 1 in, 1 out]
            n202 = Enqueue Element(queue=w414, element=cluster{string, variant} {"TreeAcessControl", variant}) -> ()  [unwired: 2 in, 3 out]
          }
          event "publish": Value Change {
            n203 = event-data() -> ()  [unwired: 1 in, 1 out]
            n204 = call <vilib>:"isConnected.vi"("error in (no error)"=w420, "Client in"=w421) -> ("error out"=w416:errorcluster, "connected"=w419:bool, "Client out"=w418:refnum<class "Client.lvclass">)  [unwired: 7 in]
            n205 = case shown="True" w419 {
              tunnel: w418 -> [w423 w429]
              tunnel: [w423 w432] -> w417
              tunnel: w416 -> [w422 w431]
              tunnel: [w422 w430] -> w415
              frame False {
              }
              frame True {
                n206 = local read "mac"() -> (w425:string)
                n207 = Format Into String(format string="esp32/access/%s", w425) -> (resulting string=w424:string)  [unwired: 2 in, 1 out]
                n208 = local read "msg"() -> (w428:string)
                n209 = String To Byte Array(string=w428) -> (unsigned byte array=w427:u8[])
                n210 = call <vilib>:"Publish (Raw Payload).vi"("error in (no error)"=w431, "Binary Payload"=w427, "Topic Name"=w424, "Client in"=w429) -> ("error out"=w430:errorcluster, "Client out"=w432:refnum<class "Client.lvclass">)  [unwired: 5 in, 1 out]
              }
            }
          }
        }
      }
      frame Error {
        n211 = local write "last error"(w435) -> ()
        n212 = Unbundle By Name(w435) -> ("code"=w439:i32)
        n213 = case shown="56, 66" w439 {
          tunnel: w438 -> [w444 w446]
          tunnel: [w444 w446] -> w440
          tunnel: w435 -> [w443 _]
          tunnel: [w443 _] -> w437
          tunnel: [TRUE _] -> w436
          tunnel: w434 -> [w441 w445]
          tunnel: [w441 w445] -> w433
          frame Default {
            # "Stop on Unhandled Error"
          }
          frame 56, 66 {
            # "Disconnected"
          }
        }
      }
    }
  }
  n214 = Unregister For Events(event registration refnum=w25) -> ()  [unwired: 1 in, 1 out]
  n215 = call <vilib>:"Stop.vi"("error in (no error)"=w32, "MQTT_Base in"=w30) -> ("error out"=w31:errorcluster, "MQTT_Base out"=w29:refnum<class "Client.lvclass">)  [unwired: 7 in, 1 out]
  n216 = call <vilib>:"Destroy.vi"("error in (no error)"=w31, "MQTT_Base in"=w29) -> ("error out"=→"last error":errorcluster)  [unwired: 8 in, 1 out]
